vi "Multi Graph Toggle.vi"(8 "error in (no error)":errorcluster, 9 "Array":bool[](array[boolean]), 10 "Waveform Chart":refnum<vi>) -> (0 "error out":errorcluster)   [LabVIEW 2009]
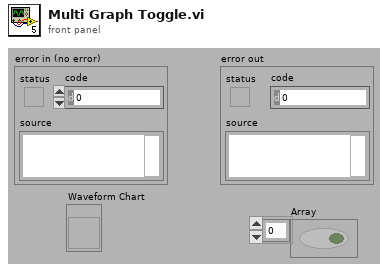
[diagram p1: front panel]
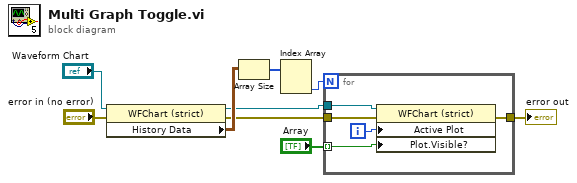
[diagram p0: block diagram]
diagram:
  n1 = property class="WFChart (strict)"(reference="Waveform Chart", error in="error in (no error)") -> (reference out=w4:refnum<vi>, error out=w5:errorcluster, "History Data"=w8:waveform(dbl)[][])
  n2 = Array Size(array=w8) -> (size(s)=w7:i32[])
  n3 = Index Array(array=w7) -> (element #2=w1:i32)  [unwired: 2 in, 1 out]
  n4 = for {
    N: w1 -> [_]
    tunnel: "Array" -> [w14] mode=indexing
    tunnel: [w12] -> w3
    tunnel: w5 -> [w11]
    tunnel: w4 -> [w10]
    i -> [w13]
    n5 = property on="Property Node" class="WFChart (strict)"(reference=w10, error in=w11, "Active Plot"=w13, "Plot.Visible?"=w14) -> (error out=w12:errorcluster)  [unwired: 1 out]
  }
  "error out" <- w3
